vi "GraphOrMap.vi"(0 "ScanCoords [mm]":T1, 1 "Order selection":u16(ring)=1 items=["X->Z->Y"=6, "Y->Z->X"=5, "Z->X->Y"=3, "Y->X->Z"=2, "Z->Y->X"=4, "X->Y->Z"=1]) -> (2 "Axis for graph":i32, 3 "3D":bool, 4 "MAP":bool)   [LabVIEW 2015]
panel:
  out "invert":bool
  out "1D":bool
  out "GRAPH":bool
  # "ustala czy dla danych parametrów skanu zastosowac mape 2D czy tez wykres:\njesli mapa 2D lub 3D wykonywana jest najpierw w kierunku Z potem X lub Y \nwyswietlony zostanie wykres (profil głębokościowy dla danego X i Y);\njesli dwa z trzech wymiarów skanu są stałe (nie dokonuje sie w nich przesuniecie)\nrównież zostanie wyswietlony wykres;\nwe wszystkich pozostalych przypadkach wyswietlana jest mapa 2D dla danej warstwy"
  # "checks how to visualise data: with plot (MAP = FALSE) or map (MAP=TRUE):\n1) if this is 2D map or 3D map where Z axis moves first it will create depth plot\n2) if the only one coordinate moves it will also grate plot instead of map"
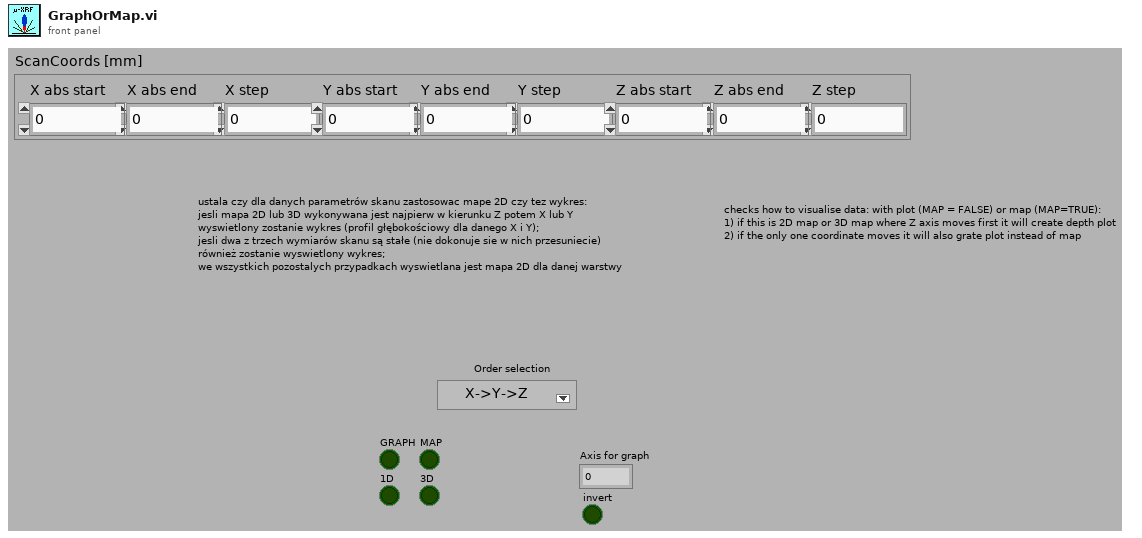
[diagram p1: front panel]
types:
  T1 = cluster{"X abs start":dbl, "X abs end":dbl, "Y abs start":dbl, "Y abs end":dbl, "Z abs start":dbl, "Z abs end":dbl, "X step":dbl, "Y step":dbl, "Z step":dbl}
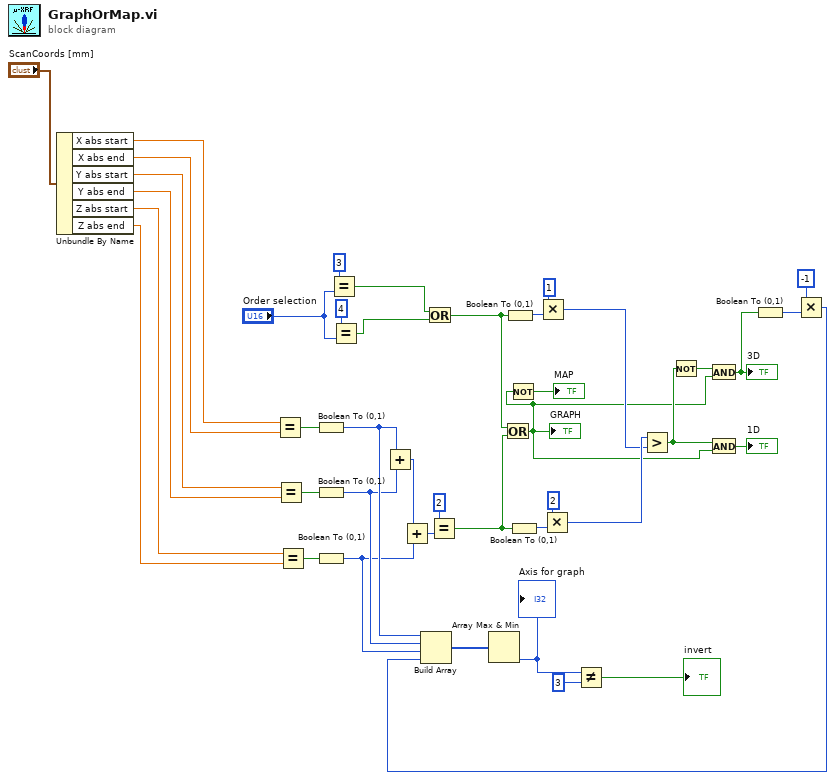
[diagram p0: block diagram]
diagram:
  n1 = Unbundle By Name("ScanCoords [mm]") -> ("X abs start"=w6:dbl, "X abs end"=w5:dbl, "Y abs start"=w4:dbl, "Y abs end"=w3:dbl, "Z abs start"=w2:dbl, "Z abs end"=w1:dbl)
  n2 = Equal?(x=w6, y=w5) -> (x = y?=w42:bool)
  n3 = Equal?(x=w4, y=w3) -> (x = y?=w41:bool)
  n4 = Equal?(x=w2, y=w1) -> (x = y?=w40:bool)
  n5 = Boolean To (0,1)(Boolean=w42) -> (0, 1=w18:i16)
  n6 = Boolean To (0,1)(Boolean=w41) -> (0, 1=w17:i16)
  n7 = Boolean To (0,1)(Boolean=w40) -> (0, 1=w16:i16)
  n8 = Equal?(x=3, y="Order selection") -> (x = y?=w33:bool)
  n9 = Equal?(x=4, y="Order selection") -> (x = y?=w32:bool)
  n10 = Add(x=w18, y=w17) -> (x+y=w39:i16)
  n11 = Add(x=w39, y=w16) -> (x+y=w38:i16)
  n12 = Or(x=w33, y=w32) -> (x .or. y?=w31:bool)
  n13 = Equal?(x=i16 2, y=w38) -> (x = y?=w26:bool)
  n14 = Or(x=w31, y=w26) -> (x .or. y?=w19:bool)
  "GRAPH" <- w19
  n15 = Boolean To (0,1)(Boolean=w31) -> (0, 1=w30:i16)
  n16 = Not(x=w19) -> (.not. x?=→"MAP":bool)
  n17 = Boolean To (0,1)(Boolean=w26) -> (0, 1=w28:i16)
  n18 = Multiply(x=i16 1, y=w30) -> (x*y=w24:i16)
  n19 = Multiply(x=i16 2, y=w28) -> (x*y=w25:i16)
  n20 = Greater?(x=w25, y=w24) -> (0:w21:bool)
  n21 = Not(x=w21) -> (.not. x?=w22:bool)
  n22 = And(x=w22, y=w19) -> (x .and. y?=w14:bool)
  "3D" <- w14
  n23 = And(x=w21, y=w19) -> (x .and. y?=→"1D":bool)
  n24 = Boolean To (0,1)(Boolean=w14) -> (0, 1=w13:i16)
  n25 = Multiply(x=i16 -1, y=w13) -> (x*y=w11:i16)
  n26 = Build Array(w18, w17, w16, w11) -> (w15:i16[])
  n27 = Array Max & Min(array=w15) -> (min index (indices)=w10:i32)  [unwired: 3 out]
  "Axis for graph" <- w10
  n28 = Not Equal?(x=w10, y=3) -> (x != y?=→"invert":bool)
